vi "RampRateMultiple.vi"(6 "return immediately":bool, 8 "error in (no error)":T1, 9 "ramp rates":dbl[](array[numeric]), 10 "axis names":string[](array[string]), 11 "controller in":refnum<k24>) -> (0 "error out":T1, 3 "controller out":refnum<k24>)   [LabVIEW 2010]
doc: "Ramp rate sets the acceleration and deceleration rates for the respective axis names."
uses:
  c:/aerotech/controller/5.xx.xxx/ensemble/pc/labview/2010/bin/Aerotech.Ensemble.dll
  bin/Aerotech.Ensemble.dll
  c:/aerotech/controller/5.xx.xxx/ensemble/pc/labview/2010/bin/Aerotech.Ensemble.LabVIEW.dll
  bin/Aerotech.Ensemble.LabVIEW.dll
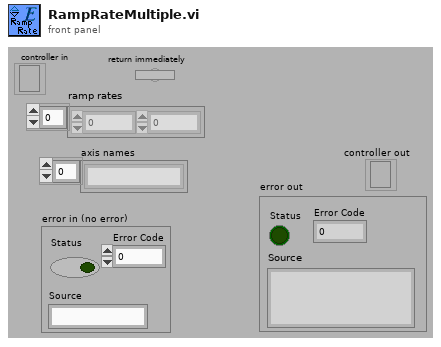
[diagram p1: front panel]
types:
  T1 = cluster{"Status":bool, "Error Code":i32, "Source":string}
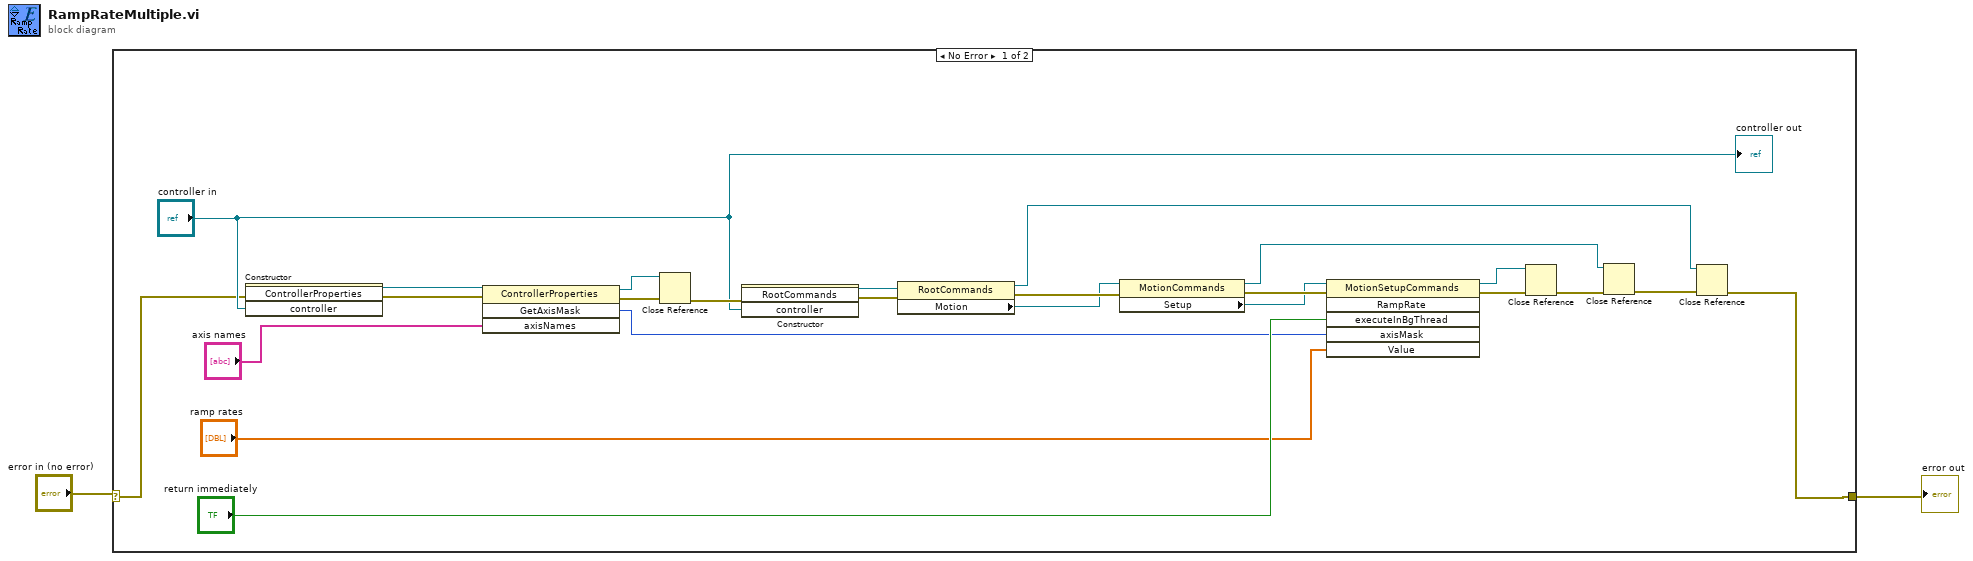
[diagram p0: block diagram]
diagram:
  n1 = case shown="No Error" "error in (no error)" {
    selector: "error in (no error)" -> [w4 w27]
    tunnel: [w3 w27] -> w1
    frame No Error {
      n2 = constructor class="ControllerProperties"(error in=w4, "controller"="controller in") -> (reference out=w25:refnum<k24>, error out=w26:errorcluster)  [unwired: 2 in, 2 out]
      n3 = invoke class="ControllerProperties" method="GetAxisMask"(reference=w25, error in=w26, "axisNames"="axis names") -> (reference out=w22:refnum<k24>, error out=w23:errorcluster, "GetAxisMask"=w7:i32)  [unwired: 1 in, 1 out]
      n4 = Close Reference(reference=w22, error in (no error)=w23) -> (error out=w21:errorcluster)
      n5 = constructor class="RootCommands"(error in=w21, "controller"="controller in") -> (reference out=w20:refnum<k24>, error out=w19:errorcluster)  [unwired: 2 in, 2 out]
      n6 = property class="RootCommands"(reference=w20, error in=w19) -> (reference out=w9:refnum<k24>, error out=w18:errorcluster, "Motion"=w17:refnum<k24>)
      n7 = property class="MotionCommands"(reference=w17, error in=w18) -> (reference out=w11:refnum<k24>, error out=w16:errorcluster, "Setup"=w15:refnum<k24>)
      n8 = invoke class="MotionSetupCommands" method="RampRate"(reference=w15, error in=w16, "executeInBgThread"="return immediately", "axisMask"=w7, "Value"="ramp rates") -> (reference out=w13:refnum<k24>, error out=w14:errorcluster)  [unwired: 1 in, 4 out]
      n9 = Close Reference(reference=w13, error in (no error)=w14) -> (error out=w12:errorcluster)
      n10 = Close Reference(reference=w11, error in (no error)=w12) -> (error out=w10:errorcluster)
      n11 = Close Reference(reference=w9, error in (no error)=w10) -> (error out=w3:errorcluster)
      "controller out" <- "controller in"
    }
    frame Error {
    }
  }
  "error out" <- w1
